vi "Focus Read Positions.vi"(8 "error in (no error)":errorcluster, 11 "NewFocus in":refnum<class "NewFocus.lvclass">) -> (0 "error out":errorcluster, 2 "Motor Positions":i32[](array[numeric]), 3 "NewFocus out":refnum<class "NewFocus.lvclass">)   [LabVIEW 2024, in "NewFocus.lvclass"]
uses:
  NewFocus.lvclass
  C:/Development/Prime-RIMAS/Focus/Focus Class/Focus Class.lvclass
  NewFocus.lvclass/NewFocus.ctl
  Focus Class/Focus Class.lvclass/Focus Class.ctl
  Focus Class/Focus Class.lvclass
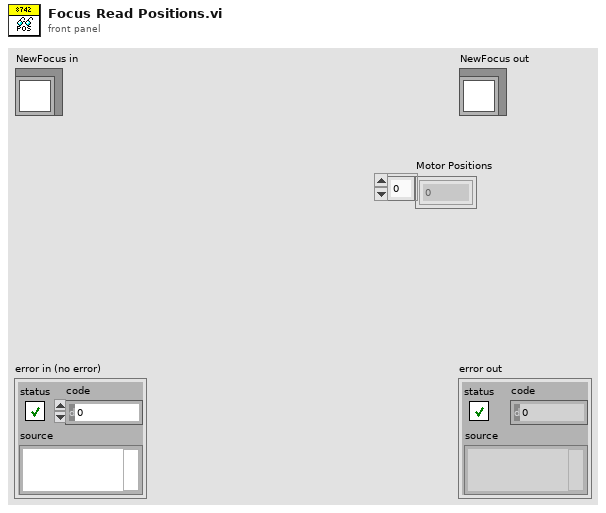
[diagram p1: front panel]
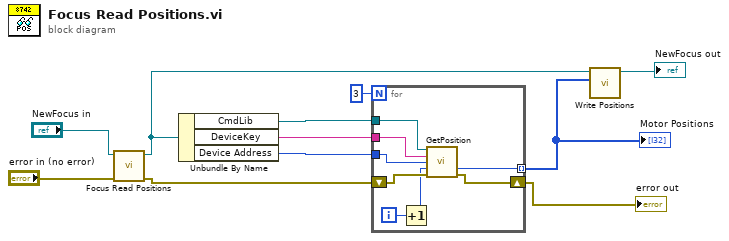
[diagram p0: block diagram]
diagram:
  n1 = call-parent "Focus Read Positions.vi"("error in (no error)"="error in (no error)", "Focus Class in"="NewFocus in") -> ("error out"=w5:errorcluster, "Focus Class out"=w3:refnum<class "NewFocus.lvclass">)  [unwired: 7 in, 1 out]
  n2 = Unbundle By Name(w3) -> ("CmdLib"=w8:refnum<k24>, "DeviceKey"=w7:string, "Device Address"=w6:i32)
  n3 = for {
    N: 3 -> [_]
    tunnel: w8 -> [w19]
    tunnel: w7 -> [w18]
    tunnel: w6 -> [w17]
    shift-right: [w14] -> w4
    shift-left: w5 -> [w15]
    tunnel: [w13] -> w1 mode=indexing
    i -> [w16]
    n4 = Increment(x=w16) -> (x+1=w12:i32)
    n5 = call "GetPosition.vi"("CmdLib In"=w19, "DeviceKey In"=w18, "Device Address In"=w17, "Motor"=w12, "error in (no error)"=w15) -> ("Position"=w13:i32, "error out"=w14:errorcluster)  [unwired: 6 in, 3 out]
  }
  "error out" <- w4
  "Motor Positions" <- w1
  n6 = call "Write Positions.vi"("Positions"=w1, "Focus Class in"=w3) -> ("Focus Class out"=→"NewFocus out":refnum<class "NewFocus.lvclass">)  [unwired: 8 in, 1 out]
